vi "Get Library Info.vi"(0 "object in":refnum<class "HPS-17000-PowerModule.lvclass">, 11 "Error In":errorcluster) -> (4 "object out":refnum<class "HPS-17000-PowerModule.lvclass">, 6 "PPL Filename":string, 8 "Build Version":string="v1.0.0.46", 15 "Error Out":errorcluster)   [LabVIEW 2023, in "HPS-17000-PowerModule.lvlib" / "HPS-17000-PowerModule.lvclass"]
uses:
  HPS-17000-PowerModule.lvclass
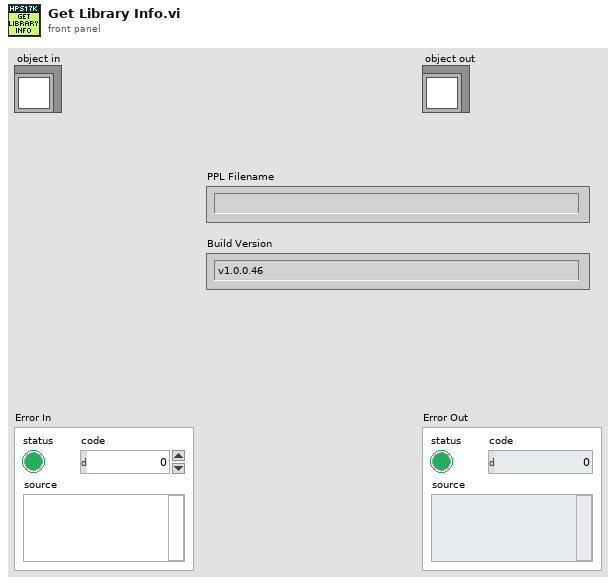
[diagram p1: front panel]
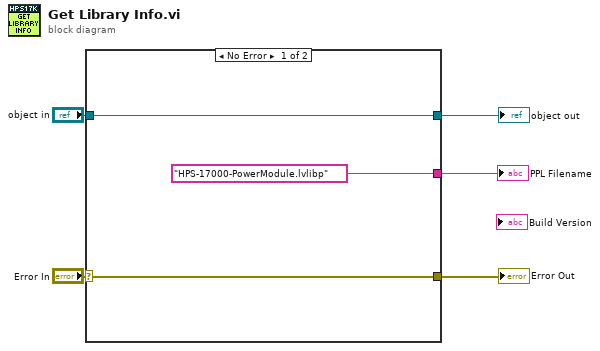
[diagram p0: block diagram]
diagram:
  n1 = case shown="No Error" "Error In" {
    selector: "Error In" -> [w7 w9]
    tunnel: ["HPS-17000-PowerModule.lvlibp" _] -> w5
    tunnel: [w7 w9] -> w4
    tunnel: [w8 w10] -> w3
    tunnel: "object in" -> [w8 w10]
    frame No Error {
    }
    frame Error {
    }
  }
  "Error Out" <- w4
  "object out" <- w3
  "PPL Filename" <- w5
